vi "Configure.vi"(8 "error in (no error)":errorcluster, 10 "measurementservice_DMMConfigRequest_Data":T3, 11 "DMMSession":refnum<k15>) -> (0 "error out":errorcluster, 2 "measurementservice_DMMConfigResponse_Data":T1)   [LabVIEW 2019, in "ctet_dmm User Library.lvlib"]
uses:
  ctet_dmm User Library.lvlib
  Servers/ctet_dmm/ctet_dmm Class/RPC Messages/measurementservice_DMMConfigRequest/measurementservice_DMMConfigRequest_Data.ctl
  Servers/ctet_dmm/ctet_dmm Class/RPC Messages/measurementservice_DMMConfigResponse/measurementservice_DMMConfigResponse_Data.ctl
  Servers/ctet_dmm/ctet_dmm Class/RPC Messages/measurementservice_ErrorOut/measurementservice_ErrorOut_Data.ctl
  <instrlib>/niDMM/nidmm.llb/niDMM Control Actions.ctl
  <instrlib>/niDMM/nidmm.llb/niDMM Configure Measurement Digits.vi
  Servers/ctet_dmm/ctet_dmm Class/ctet_dmm.lvclass
panel:
  in  "DMM Function Array":i32[](array[numeric])=[1, 2, 3, 4, 5, 101, 1002, 104, 105, 1001, 1005, 1006, 108]
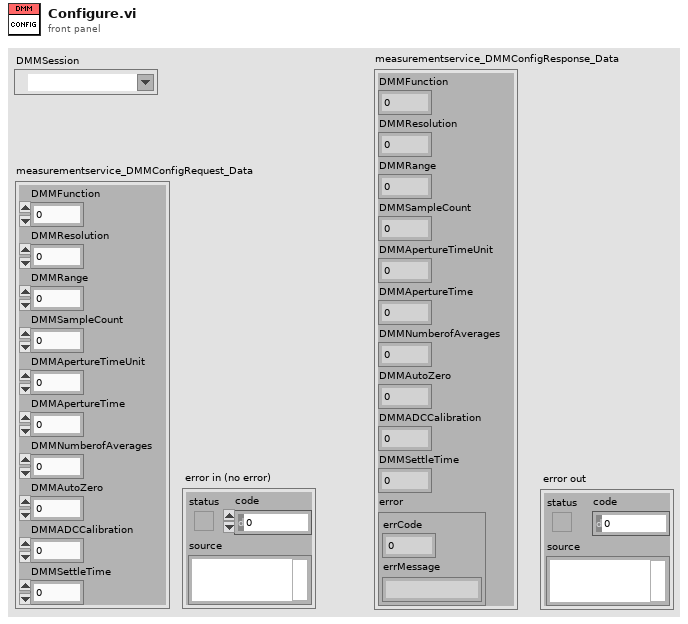
[diagram p1: front panel]
types:
  T1 = typedef "ctet_dmm.lvlib/ctet_dmm.lvclass/measurementservice_DMMConfigResponse_Data.ctl" = cluster{"DMMFunction":i64, "DMMResolution":dbl, "DMMRange":dbl, "DMMSampleCount":i64, "DMMApertureTimeUnit":i64, "DMMApertureTime":dbl, "DMMNumberofAverages":i64, "DMMAutoZero":i64, "DMMADCCalibration":i64, "DMMSettleTime":dbl, "error":T2}
  T2 = typedef "ctet_dmm.lvlib/ctet_dmm.lvclass/measurementservice_ErrorOut_Data.ctl" = cluster{"errCode":i64, "errMessage":string}
  T3 = typedef "ctet_dmm.lvlib/ctet_dmm.lvclass/measurementservice_DMMConfigRequest_Data.ctl" = cluster{"DMMFunction":i64, "DMMResolution":dbl, "DMMRange":dbl, "DMMSampleCount":i64, "DMMApertureTimeUnit":i64, "DMMApertureTime":dbl, "DMMNumberofAverages":i64, "DMMAutoZero":i64, "DMMADCCalibration":i64, "DMMSettleTime":dbl}
  T4 = typedef "niDMM Control Actions.ctl" = i32
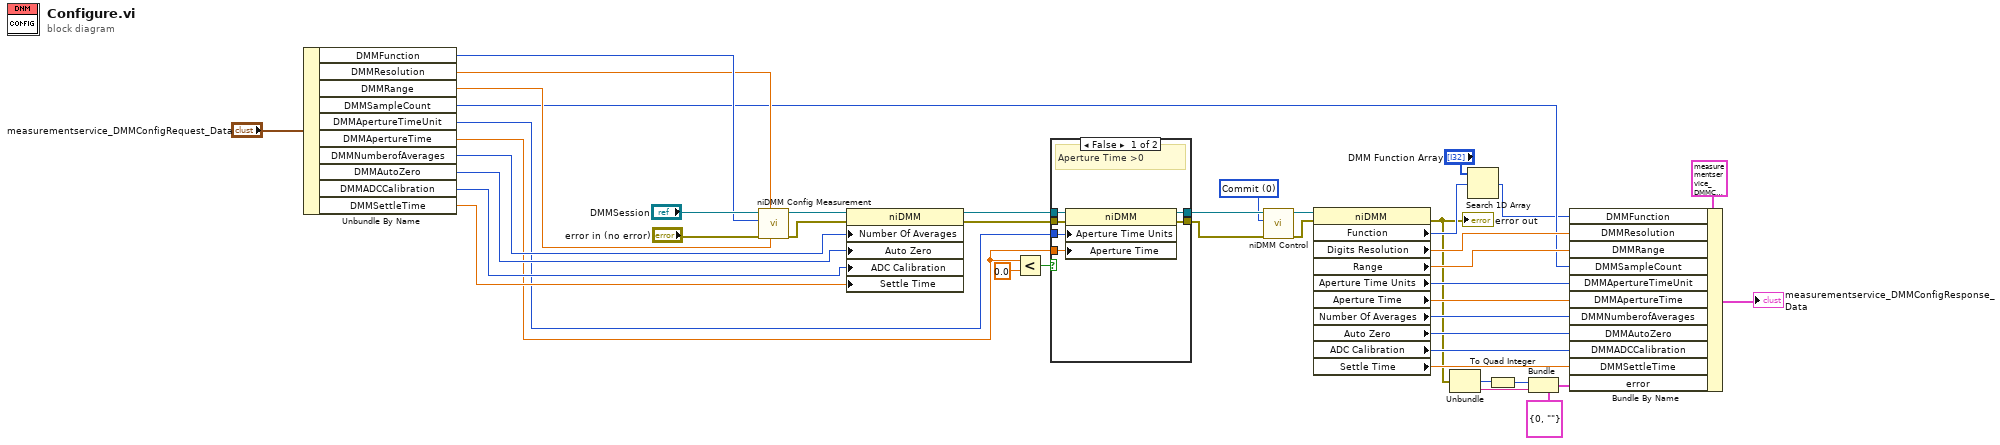
[diagram p0: block diagram]
diagram:
  w25 = T4 0 items=["Commit"] ("Control Action")
  n1 = Unbundle By Name("measurementservice_DMMConfigRequest_Data") -> ("DMMFunction"=w42:i64, "DMMResolution"=w41:dbl, "DMMRange"=w40:dbl, "DMMSampleCount"=w14:i64, "DMMApertureTimeUnit"=w29:i64, "DMMApertureTime"=w28:dbl, "DMMNumberofAverages"=w37:i64, "DMMAutoZero"=w36:i64, "DMMADCCalibration"=w35:i64, "DMMSettleTime"=w34:dbl)
  n2 = call-poly <instrlib>:"niDMM Config Measurement.vi"("Range"=w40, "Resolution in Digits"=w41, "error in (no error)"="error in (no error)", "Function"=w42, "instrument handle"="DMMSession") -> ("error out"=w38:errorcluster, "instrument handle out"=w39:refnum<k15>)  [unwired: 5 in]
  n3 = property class="niDMM"(reference=w39, error in=w38, "Number Of Averages"=w37, "Auto Zero"=w36, "ADC Calibration"=w35, "Settle Time"=w34) -> (reference out=w33:refnum<k15>, error out=w32:errorcluster)
  n4 = Less?(x=w28, y=0.0 ("Configuration:Advanced:Aperture Time")) -> (x < y?=w30:bool)
  n5 = case shown="False" w30 {
    tunnel: w33 -> [w49 w51]
    tunnel: w32 -> [w48 w50]
    tunnel: [w47 w51] -> w27
    tunnel: [w46 w50] -> w26
    tunnel: w29 -> [w45 _]
    tunnel: w28 -> [w44 _]
    frame False {
      # "Aperture Time >0"
      n6 = property class="niDMM"(reference=w49, error in=w48, "Aperture Time Units"=w45, "Aperture Time"=w44) -> (reference out=w47:refnum<k15>, error out=w46:errorcluster)
    }
    frame True {
      # "Aperture Time <0"
    }
  }
  n7 = call <instrlib>:"niDMM Control.vi"("error in (no error)"=w26, "Control Action"=w25, "instrument handle"=w27) -> ("error out"=w23:errorcluster, "instrument handle out"=w24:refnum<k15>)  [unwired: 7 in]
  n8 = property class="niDMM"(reference=w24, error in=w23) -> (error out=w7:errorcluster, "Function"=w12:i32, "Digits Resolution"=w15:dbl, "Range"=w16:dbl, "Aperture Time Units"=w17:i32, "Aperture Time"=w18:dbl, "Number Of Averages"=w19:i32, "Auto Zero"=w20:i32, "ADC Calibration"=w21:i32, "Settle Time"=w22:dbl)  [unwired: 1 out]
  "error out" <- w7
  n9 = Unbundle(w7) -> ("code"=w3:i32, "source"=w9:string)  [unwired: 1 out]
  n10 = Search 1D Array(1D array="DMM Function Array", element=w12) -> (index of element=w11:i32)  [unwired: 1 in]
  n11 = To Quad Integer(1:w3) -> (0:w2:i64)
  n12 = Bundle(cluster=T2 {"errCode"=0, "errMessage"=""} ("error"), "errCode"=w2, "errMessage"=w9) -> (w10:T2)
  n13 = Bundle By Name(cluster=T1 {"DMMFunction"=0, "DMMResolution"=0.0, "DMMRange"=0.0, "DMMSampleCount"=0, "DMMApertureTimeUnit"=0, "DMMApertureTime"=0.0, "DMMNumberofAverages"=0, "DMMAutoZero"=0, "DMMADCCalibration"=0, "DMMSettleTime"=0.0, "error"={"errCode"=0, "errMessage"=""}} ("measurementservice_DMMConfigResponse_Data"), "DMMFunction"=w11, "DMMResolution"=w15, "DMMRange"=w16, "DMMSampleCount"=w14, "DMMApertureTimeUnit"=w17, "DMMApertureTime"=w18, "DMMNumberofAverages"=w19, "DMMAutoZero"=w20, "DMMADCCalibration"=w21, "DMMSettleTime"=w22, "error"=w10) -> (→"measurementservice_DMMConfigResponse_Data":T1)
